vi "MDAQ_SaveTime.vi"(9 "Cluster In":T1 {"CV"."Temperature Array" scale=0.0..100.0}, 10 "Status_Cluster":T3 {"GATESTOP" format="%04x"; "GATESTRT" format="%04x"; "AMPLITUDE" format="%04x"; "M_CYCLES" format="%04x"; "N_CYCLES" format="%04x"; "STEP" format="%04x"; "BASE" format="%04x"; "CHAN" format="%04x"}) -> (1 "Cluster Out":T1 {"CV"."Temperature Array" scale=0.0..100.0}, 2 "Status_Cluster Out":T3 {"GATESTOP" format="%04x"; "GATESTRT" format="%04x"; "AMPLITUDE" format="%04x"; "M_CYCLES" format="%04x"; "N_CYCLES" format="%04x"; "STEP" format="%04x"; "BASE" format="%04x"; "CHAN" format="%04x"})   [LabVIEW 2021]
uses:
  Status_Cluster.ctl
  GUI_Def.ctl
  Mode_Enum.ctl
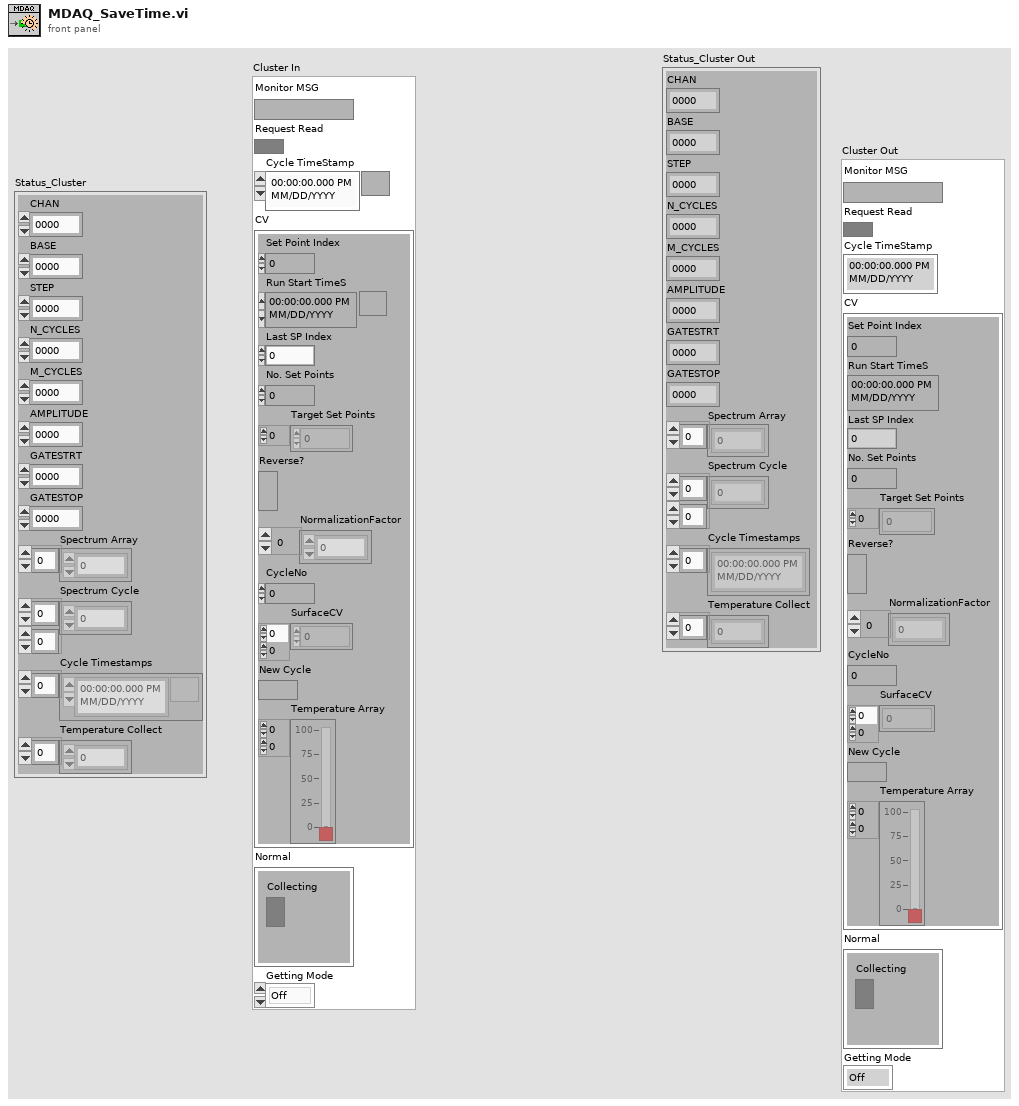
[diagram p1: front panel]
types:
  T1 = typedef "GUI_Def.ctl" = cluster{"Monitor MSG":string, "Request Read":bool, "Cycle TimeStamp":timestamp, "CV":cluster{"Set Point Index":u32, "Run Start TimeS":timestamp, "Last SP Index":u32, "No. Set Points":u32, "Target Set Points":i32[], "Reverse?":bool, "NormalizationFactor":i32[], "CycleNo":i32, "SurfaceCV":dbl[][], "New Cycle":bool, "Temperature Array":dbl[][]}, "Normal":cluster{"Collecting":bool}, "Getting Mode":T2}
  T2 = typedef "Mode_Enum.ctl" = enum16{"Off", "Normal", "CV+Temp", "CV"}
  T3 = typedef "Status_Cluster.ctl" = cluster{"CHAN":u32, "BASE":u32, "STEP":u32, "N_CYCLES":u32, "M_CYCLES":u32, "AMPLITUDE":u32, "GATESTRT":u32, "GATESTOP":u32, "Spectrum Array":u32[], "Spectrum Cycle":u32[][], "Cycle Timestamps":timestamp[], "Temperature Collect":dbl[]}
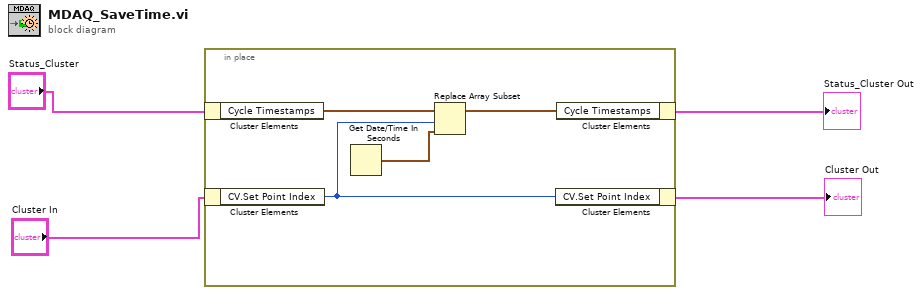
[diagram p0: block diagram]
diagram:
  n1 = in-place {
    n2 = in-place-cluster #1("Status_Cluster") -> ("Cycle Timestamps"=w8:timestamp[])
    n3 = in-place-cluster #2("Cluster In") -> ("CV.Set Point Index"=w5:u32)
    n4 = Get Date/Time In Seconds() -> (seconds since 1Jan1904=w7:timestamp)
    n5 = Replace Array Subset(array=w8, new element=w7, index=w5) -> (w6:timestamp[])
    n6 = in-place-cluster #2("CV.Set Point Index"=w5) -> (→"Cluster Out":T1)
    n7 = in-place-cluster #1("Cycle Timestamps"=w6) -> (→"Status_Cluster Out":T3)
  }
